vi "VHT Subcarrier to Frequency Offset Index.vi"(8 "primary channel selector":fxp<+,2,0>, 9 "bandwidth":enum16{"20MHz", "40MHz", "80MHz"}(ring), 10 "subcarrier index":u8) -> (1 "frequency offset index":fxp<+/-,9,9>, 2 "first non-HT subband":fxp<+,2,2>)   [LabVIEW 2020]
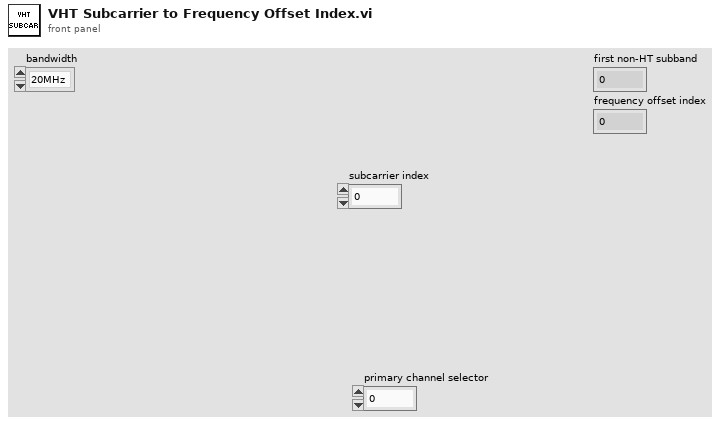
[diagram p1: front panel]
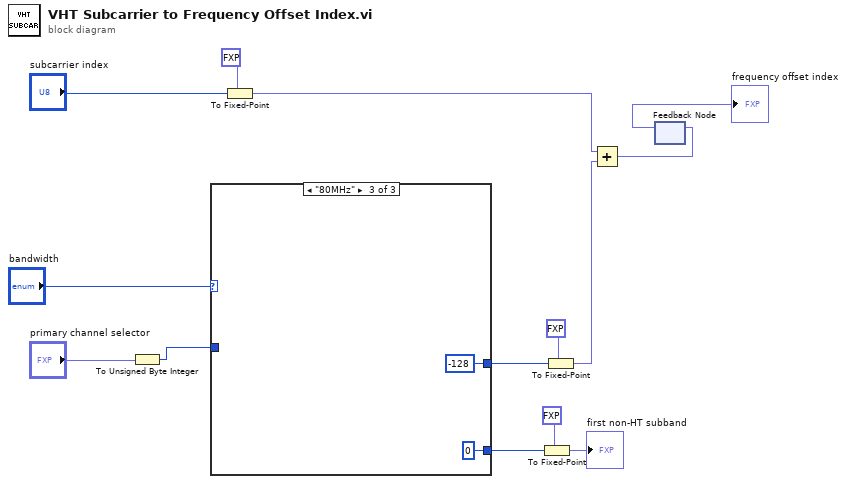
[diagram p0: block diagram]
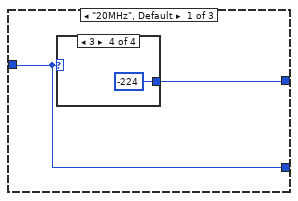
[diagram p2: hidden frame]
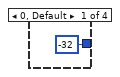
[diagram p3: hidden frame]
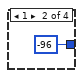
[diagram p4: hidden frame]
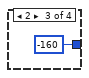
[diagram p5: hidden frame]
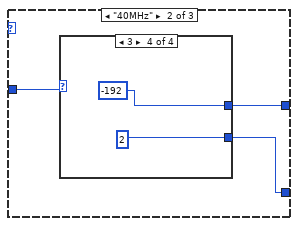
[diagram p6: hidden frame]
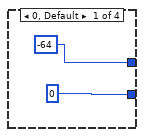
[diagram p7: hidden frame]
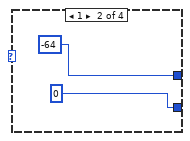
[diagram p8: hidden frame]
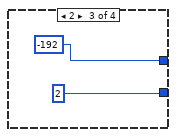
[diagram p9: hidden frame]
diagram:
  n1 = To Unsigned Byte Integer(number="primary channel selector") -> (unsigned 8bit integer=w10:u8)
  n2 = case shown="\"80MHz\"" "bandwidth" {
    tunnel: w10 -> [w16 w23 _]
    tunnel: [w15 w22 i16 -128] -> w8
    tunnel: [w16 w21 u8 0] -> w6
    frame "20MHz", Default {
      n3 = case shown="3" w16 {
        tunnel: [i16 -32 i16 -96 i16 -160 i16 -224] -> w15
        frame 0, Default {
        }
        frame 1 {
        }
        frame 2 {
        }
        frame 3 {
        }
      }
    }
    frame "40MHz" {
      n4 = case shown="3" w23 {
        tunnel: [i16 -64 i16 -64 i16 -192 i16 -192] -> w22
        tunnel: [u8 0 u8 0 u8 2 u8 2] -> w21
        frame 0, Default {
        }
        frame 1 {
        }
        frame 2 {
        }
        frame 3 {
        }
      }
    }
    frame "80MHz" {
    }
  }
  n5 = To Fixed-Point(fixed-point type=fxp<+,8,8> 0.0, number="subcarrier index") -> (fixed-point=w4:fxp<+,8,8>)
  n6 = To Fixed-Point(fixed-point type=fxp<+,2,2> 0.0, number=w6) -> (fixed-point=→"first non-HT subband":fxp<+,2,2>)
  n7 = To Fixed-Point(fixed-point type=fxp<+/-,16,16> 0.0, number=w8) -> (fixed-point=w3:fxp<+/-,16,16>)
  n8 = Add(x=w4, y=w3) -> (x+y=w2:fxp<+/-,9,9>)
  n9 = feedback-in #1(w2) -> ()
  n10 = feedback #1() -> (→"frequency offset index":fxp<+/-,9,9>)  [unwired: 1 in]
